vi "Util_GetLibraryVersion.vi"() -> (2 "TrajLibVersion":string)   [LabVIEW 2019, in "Trajectory_Library.lvlib"]
doc: "Return the library Trajectory Library version string.\n\n\n\nCopyright (c) 2020 James A. Simpson\nAll rights reserved.\n\nRedistribution and use in source and binary forms, with or without\nmodification, are permitted provided that the following conditions are met:\n * Redistributions of source code must retain the above copyright\n notice, this list of conditions and the following disclaimer.\n * Redistributions in binary form must reproduce the above copyright\n notice, this list of conditions and the following disclaimer in the\n documentation and/or other materials provided with the distribution.\n * Neither the name of the authors nor the\n names of its contributors may be used to endorse or promote products\n derived from this software without specific prior written permission.\n\nTHIS SOFTWARE IS PROVIDED BY THE AUTHOR AND CONTRIBUTORS``AS IS'' AND ANY\nEXPRESS OR IMPLIED WARRANTIES, INCLUDING, BUT NOT LIMITED TO, THE IMPLIED\nWARRANTIES OF MERCHANTABILITY NONINFRINGEMENT AND FITNESS FOR A PARTICULAR\nPURPOSE ARE DISCLAIMED. IN NO EVENT SHALL AUTHORS OR CONTRIBUTORS BE LIABLE FOR\nANY DIRECT, INDIRECT, INCIDENTAL, SPECIAL, EXEMPLARY, OR CONSEQUENTIAL DAMAGES\n(INCLUDING, BUT NOT LIMITED TO, PROCUREMENT OF SUBSTITUTE GOODS OR SERVICES;\nLOSS OF USE, DATA, OR PROFITS; OR BUSINESS INTERRUPTION) HOWEVER CAUSED AND\nON ANY THEORY OF LIABILITY, WHETHER IN CONTRACT, STRICT LIABILITY, OR TORT\n(INCLUDING NEGLIGENCE OR OTHERWISE) ARISING IN ANY WAY OUT OF THE USE OF THIS\nSOFTWARE, EVEN IF ADVISED OF THE POSSIBILITY OF SUCH DAMAGE.\n\n---------------------------------------------------------------------------------------------------\n==============================================================================\nCopyrights and Licenses for Third Party Software Distributed with FRC LV TRAJECTORY LIbrary\n==============================================================================\nThe FRC LV Trajectory Library software contains code written by and derived from \nthird parties. The copyrights, license, and restrictions which apply to each piece \nof software is included later in this file and/or inside of the individual \napplicable source files.\n\nThe disclaimer of warranty in the FRC LV Trajectory Library license above applies \nto all code in FRC LV Trajectory Library, and nothing in any of the other licenses \ngives permission to use the names of FIRST nor the names of the FRC LV Trajectory \nLibrary contributors to endorse or promote products derived from this software.\n\nThe following pieces of software have additional or alternate copyrights,\nlicenses, and/or restrictions:\n\nProgram Locations\n------- ---------\nWPILIB LabVIEW code derived from WPILIB\nRoboRIO Libraries ni-libraries\nPathfinder Pathfinder Library\nJSON for Modern C++ LabVIEW code derived from WPILIB routines\nTeam 254 Library LabVIEW code derived from WPILIB SplineParameterizer.java, \n TrajectoryParameterizer.java\n\n==============================================================================\nWPILIB License\n==============================================================================\nCopyright (c) 2009-2018 FIRST\nAll rights reserved.\n\nRedistribution and use in source and binary forms, with or without\nmodification, are permitted provided that the following conditions are met:\n * Redistributions of source code must retain the above copyright\n notice, this list of conditions and the following disclaimer.\n * Redistributions in binary form must reproduce the above copyright\n notice, this list of conditions and the following disclaimer in the\n documentation and/or other materials provided with the distribution.\n * Neither the name of the FIRST nor the\n names of its contributors may be used to endorse or promote products\n derived from this software without specific prior written permission.\n\nTHIS SOFTWARE IS PROVIDED BY FIRST AND CONTRIBUTORS``AS IS'' AND ANY\nEXPRESS OR IMPLIED WARRANTIES, INCLUDING, BUT NOT LIMITED TO, THE IMPLIED\nWARRANTIES OF MERCHANTABILITY NONINFRINGEMENT AND FITNESS FOR A PARTICULAR\nPURPOSE ARE DISCLAIMED. IN NO EVENT SHALL FIRST OR CONTRIBUTORS BE LIABLE FOR\nANY DIRECT, INDIRECT, INCIDENTAL, SPECIAL, EXEMPLARY, OR CONSEQUENTIAL DAMAGES\n(INCLUDING, BUT NOT LIMITED TO, PROCUREMENT OF SUBSTITUTE GOODS OR SERVICES;\nLOSS OF USE, DATA, OR PROFITS; OR BUSINESS INTERRUPTION) HOWEVER CAUSED AND\nON ANY THEORY OF LIABILITY, WHETHER IN CONTRACT, STRICT LIABILITY, OR TORT\n(INCLUDING NEGLIGENCE OR OTHERWISE) ARISING IN ANY WAY OUT OF THE USE OF THIS\nSOFTWARE, EVEN IF ADVISED OF THE POSSIBILITY OF SUCH DAMAGE.\n\n==============================================================================\nPATHFINDER License\n==============================================================================\nThe MIT License (MIT)\n\nCopyright (c) 2016 Jaci R\n\nPermission is hereby granted, free of charge, to any person obtaining a copy\nof this software and associated documentation files (the \"Software\"), to deal\nin the Software without restriction, including without limitation the rights\nto use, copy, modify, merge, publish, distribute, sublicense, and/or sell\ncopies of the Software, and to permit persons to whom the Software is\nfurnished to do so, subject to the following conditions:\n\nThe above copyright notice and this permission notice shall be included in all\ncopies or substantial portions of the Software.\n\nTHE SOFTWARE IS PROVIDED \"AS IS\", WITHOUT WARRANTY OF ANY KIND, EXPRESS OR\nIMPLIED, INCLUDING BUT NOT LIMITED TO THE WARRANTIES OF MERCHANTABILITY,\nFITNESS FOR A PARTICULAR PURPOSE AND NONINFRINGEMENT. IN NO EVENT SHALL THE\nAUTHORS OR COPYRIGHT HOLDERS BE LIABLE FOR ANY CLAIM, DAMAGES OR OTHER\nLIABILITY, WHETHER IN AN ACTION OF CONTRACT, TORT OR OTHERWISE, ARISING FROM,\nOUT OF OR IN CONNECTION WITH THE SOFTWARE OR THE USE OR OTHER DEALINGS IN THE\nSOFTWARE.\n\n==============================================================================\nJSON for Modern C++ License\n==============================================================================\n\n __ _____ _____ _____\n __| | __| | | | JSON for Modern C++\n| | |__ | | | | | | version 2.1.1\n|_____|_____|_____|_|___| https://github.com/nlohmann/json\n\nLicensed under the MIT License <http://opensource.org/licenses/MIT>.\nCopyright (c) 2013-2017 Niels Lohmann <http://nlohmann.me>.\n\nPermission is hereby granted, free of charge, to any person obtaining a copy\nof this software and associated documentation files (the \"Software\"), to deal\nin the Software without restriction, including without limitation the rights\nto use, copy, modify, merge, publish, distribute, sublicense, and/or sell\ncopies of the Software, and to permit persons to whom the Software is\nfurnished to do so, subject to the following conditions:\n\nThe above copyright notice and this permission notice shall be included in all\ncopies or substantial portions of the Software.\n\nTHE SOFTWARE IS PROVIDED \"AS IS\", WITHOUT WARRANTY OF ANY KIND, EXPRESS OR\nIMPLIED, INCLUDING BUT NOT LIMITED TO THE WARRANTIES OF MERCHANTABILITY,\nFITNESS FOR A PARTICULAR PURPOSE AND NONINFRINGEMENT. IN NO EVENT SHALL THE\nAUTHORS OR COPYRIGHT HOLDERS BE LIABLE FOR ANY CLAIM, DAMAGES OR OTHER\nLIABILITY, WHETHER IN AN ACTION OF CONTRACT, TORT OR OTHERWISE, ARISING FROM,\nOUT OF OR IN CONNECTION WITH THE SOFTWARE OR THE USE OR OTHER DEALINGS IN THE\nSOFTWARE.\n\n\n\n\n================\nTeam 254 Library\n================\nMIT License\n\nCopyright (c) 2018 Team 254\n\nPermission is hereby granted, free of charge, to any person obtaining a copy\nof this software and associated documentation files (the \"Software\"), to deal\nin the Software without restriction, including without limitation the rights\nto use, copy, modify, merge, publish, distribute, sublicense, and/or sell\ncopies of the Software, and to permit persons to whom the Software is\nfurnished to do so, subject to the following conditions:\n\nThe above copyright notice and this permission notice shall be included in all\ncopies or substantial portions of the Software.\n\nTHE SOFTWARE IS PROVIDED \"AS IS\", WITHOUT WARRANTY OF ANY KIND, EXPRESS OR\nIMPLIED, INCLUDING BUT NOT LIMITED TO THE WARRANTIES OF MERCHANTABILITY,\nFITNESS FOR A PARTICULAR PURPOSE AND NONINFRINGEMENT. IN NO EVENT SHALL THE\nAUTHORS OR COPYRIGHT HOLDERS BE LIABLE FOR ANY CLAIM, DAMAGES OR OTHER\nLIABILITY, WHETHER IN AN ACTION OF CONTRACT, TORT OR OTHERWISE, ARISING FROM,\nOUT OF OR IN CONNECTION WITH THE SOFTWARE OR THE USE OR OTHER DEALINGS IN THE\nSOFTWARE."
uses:
  Trajectory_Library.lvlib
panel:
  # "Copyright (c) 2020 James A. Simpson\nAll rights reserved.\n\nRedistribution and use in source and binary forms, with or without\nmodification, are permitted provided that the following conditions are met:\n    * Redistributions of source code must retain the above copyright\n      notice, this list of conditions and the following disclaimer.\n    * Redistributions in binary form must reproduce the above copyright\n      notice, this list of conditions and the following disclaimer in the\n      documentation and/or other materials provided with the distribution.\n    * Neither the name of the authors nor the\n      names of its contributors may be used to endorse or promote products\n      derived from this software without specific prior written permission.\n\nTHIS SOFTWARE IS PROVIDED BY THE AUTHOR AND CONTRIBUTORS``AS IS'' AND ANY\nEXPRESS OR IMPLIED WARRANTIES, INCLUDING, BUT NOT LIMITED TO, THE IMPLIED\nWARRANTIES OF MERCHANTABILITY NONINFRINGEMENT AND FITNESS FOR A PARTICULAR\nPURPOSE ARE DISCLAIMED. IN NO EVENT SHALL AUTHORS OR CONTRIBUTORS BE LIABLE FOR\nANY DIRECT, INDIRECT, INCIDENTAL, SPECIAL, EXEMPLARY, OR CONSEQUENTIAL DAMAGES\n(INCLUDING, BUT NOT LIMITED TO, PROCUREMENT OF SUBSTITUTE GOODS OR SERVICES;\nLOSS OF USE, DATA, OR PROFITS; OR BUSINESS INTERRUPTION) HOWEVER CAUSED AND\nON ANY THEORY OF LIABILITY, WHETHER IN CONTRACT, STRICT LIABILITY, OR TORT\n(INCLUDING NEGLIGENCE OR OTHERWISE) ARISING IN ANY WAY OUT OF THE USE OF THIS\nSOFTWARE, EVEN IF ADVISED OF THE POSSIBILITY OF SUCH DAMAGE.\n\n---------------------------------------------------------------------------------------------------\n==============================================================================\nCopyrights and Licenses for Third Party Software Distributed with FRC LV TRAJECTORY LIbrary\n==============================================================================\nThe FRC LV Trajectory Library software contains code written by and derived from \nthird parties.  The copyrights, license, and restrictions which apply to each piece \nof software is included later in this file and/or inside of the individual \napplicable source files.\n\nThe disclaimer of warranty in the FRC LV Trajectory Library license above applies \nto all code in FRC LV Trajectory Library, and nothing in any of the other licenses \ngives permission to use the names of FIRST nor the names of the FRC LV Trajectory \nLibrary contributors to endorse or promote products derived from this software.\n\nThe following pieces of software have additional or alternate copyrights,\nlicenses, and/or restrictions:\n\nProgram               Locations\n-------               ---------\nWPILIB                LabVIEW code derived from WPILIB\nRoboRIO Libraries     ni-libraries\nPathfinder            Pathfinder Library\nJSON for Modern C++   LabVIEW code derived from WPILIB routines\nTeam 254 Library      LabVIEW code derived from WPILIB SplineParameterizer.java, \n                      TrajectoryParameterizer.java\n\n==============================================================================\nWPILIB License\n==============================================================================\nCopyright (c) 2009-2018 FIRST\nAll rights reserved.\n\nRedistribution and use in source and binary forms, with or without\nmodification, are permitted provided that the following conditions are met:\n    * Redistributions of source code must retain the above copyright\n      notice, this list of conditions and the following disclaimer.\n    * Redistributions in binary form must reproduce the above copyright\n      notice, this list of conditions and the following disclaimer in the\n      documentation and/or other materials provided with the distribution.\n    * Neither the name of the FIRST nor the\n      names of its contributors may be used to endorse or promote products\n      derived from this software without specific prior written permission.\n\nTHIS SOFTWARE IS PROVIDED BY FIRST AND CONTRIBUTORS``AS IS'' AND ANY\nEXPRESS OR IMPLIED WARRANTIES, INCLUDING, BUT NOT LIMITED TO, THE IMPLIED\nWARRANTIES OF MERCHANTABILITY NONINFRINGEMENT AND FITNESS FOR A PARTICULAR\nPURPOSE ARE DISCLAIMED. IN NO EVENT SHALL FIRST OR CONTRIBUTORS BE LIABLE FOR\nANY DIRECT, INDIRECT, INCIDENTAL, SPECIAL, EXEMPLARY, OR CONSEQUENTIAL DAMAGES\n(INCLUDING, BUT NOT LIMITED TO, PROCUREMENT OF SUBSTITUTE GOODS OR SERVICES;\nLOSS OF USE, DATA, OR PROFITS; OR BUSINESS INTERRUPTION) HOWEVER CAUSED AND\nON ANY THEORY OF LIABILITY, WHETHER IN CONTRACT, STRICT LIABILITY, OR TORT\n(INCLUDING NEGLIGENCE OR OTHERWISE) ARISING IN ANY WAY OUT OF THE USE OF THIS\nSOFTWARE, EVEN IF ADVISED OF THE POSSIBILITY OF SUCH DAMAGE.\n\n==============================================================================\nPATHFINDER License\n==============================================================================\nThe MIT License (MIT)\n\nCopyright (c) 2016 Jaci R\n\nPermission is hereby granted, free of charge, to any person obtaining a copy\nof this software and associated documentation files (the \"Software\"), to deal\nin the Software without restriction, including without limitation the rights\nto use, copy, modify, merge, publish, distribute, sublicense, and/or sell\ncopies of the Software, and to permit persons to whom the Software is\nfurnished to do so, subject to the following conditions:\n\nThe above copyright notice and this permission notice shall be included in all\ncopies or substantial portions of the Software.\n\nTHE SOFTWARE IS PROVIDED \"AS IS\", WITHOUT WARRANTY OF ANY KIND, EXPRESS OR\nIMPLIED, INCLUDING BUT NOT LIMITED TO THE WARRANTIES OF MERCHANTABILITY,\nFITNESS FOR A PARTICULAR PURPOSE AND NONINFRINGEMENT. IN NO EVENT SHALL THE\nAUTHORS OR COPYRIGHT HOLDERS BE LIABLE FOR ANY CLAIM, DAMAGES OR OTHER\nLIABILITY, WHETHER IN AN ACTION OF CONTRACT, TORT OR OTHERWISE, ARISING FROM,\nOUT OF OR IN CONNECTION WITH THE SOFTWARE OR THE USE OR OTHER DEALINGS IN THE\nSOFTWARE.\n\n==============================================================================\nJSON for Modern C++ License\n==============================================================================\n\n    __ _____ _____ _____\n __|  |   __|     |   | |  JSON for Modern C++\n|  |  |__   |  |  | | | |  version 2.1.1\n|_____|_____|_____|_|___|  https://github.com/nlohmann/json\n\nLicensed under the MIT License <http://opensource.org/licenses/MIT>.\nCopyright (c) 2013-2017 Niels Lohmann <http://nlohmann.me>.\n\nPermission is hereby  granted, free of charge, to any  person obtaining a copy\nof this software and associated  documentation files (the \"Software\"), to deal\nin the Software  without restriction, including without  limitation the rights\nto  use, copy,  modify, merge,  publish, distribute,  sublicense, and/or  sell\ncopies  of  the Software,  and  to  permit persons  to  whom  the Software  is\nfurnished to do so, subject to the following conditions:\n\nThe above copyright notice and this permission notice shall be included in all\ncopies or substantial portions of the Software.\n\nTHE SOFTWARE  IS PROVIDED \"AS  IS\", WITHOUT WARRANTY  OF ANY KIND,  EXPRESS OR\nIMPLIED,  INCLUDING BUT  NOT  LIMITED TO  THE  WARRANTIES OF  MERCHANTABILITY,\nFITNESS FOR  A PARTICULAR PURPOSE AND  NONINFRINGEMENT. IN NO EVENT  SHALL THE\nAUTHORS  OR COPYRIGHT  HOLDERS  BE  LIABLE FOR  ANY  CLAIM,  DAMAGES OR  OTHER\nLIABILITY, WHETHER IN AN ACTION OF  CONTRACT, TORT OR OTHERWISE, ARISING FROM,\nOUT OF OR IN CONNECTION WITH THE SOFTWARE  OR THE USE OR OTHER DEALINGS IN THE\nSOFTWARE.\n\n\n\n\n================\nTeam 254 Library\n================\nMIT License\n\nCopyright (c) 2018 Team 254\n\nPermission is hereby granted, free of charge, to any person obtaining a copy\nof this software and associated documentation files (the \"Software\"), to deal\nin the Software without restriction, including without limitation the rights\nto use, copy, modify, merge, publish, distribute, sublicense, and/or sell\ncopies of the Software, and to permit persons to whom the Software is\nfurnished to do so, subject to the following conditions:\n\nThe above copyright notice and this permission notice shall be included in all\ncopies or substantial portions of the Software.\n\nTHE SOFTWARE IS PROVIDED \"AS IS\", WITHOUT WARRANTY OF ANY KIND, EXPRESS OR\nIMPLIED, INCLUDING BUT NOT LIMITED TO THE WARRANTIES OF MERCHANTABILITY,\nFITNESS FOR A PARTICULAR PURPOSE AND NONINFRINGEMENT. IN NO EVENT SHALL THE\nAUTHORS OR COPYRIGHT HOLDERS BE LIABLE FOR ANY CLAIM, DAMAGES OR OTHER\nLIABILITY, WHETHER IN AN ACTION OF CONTRACT, TORT OR OTHERWISE, ARISING FROM,\nOUT OF OR IN CONNECTION WITH THE SOFTWARE OR THE USE OR OTHER DEALINGS IN THE\nSOFTWARE."
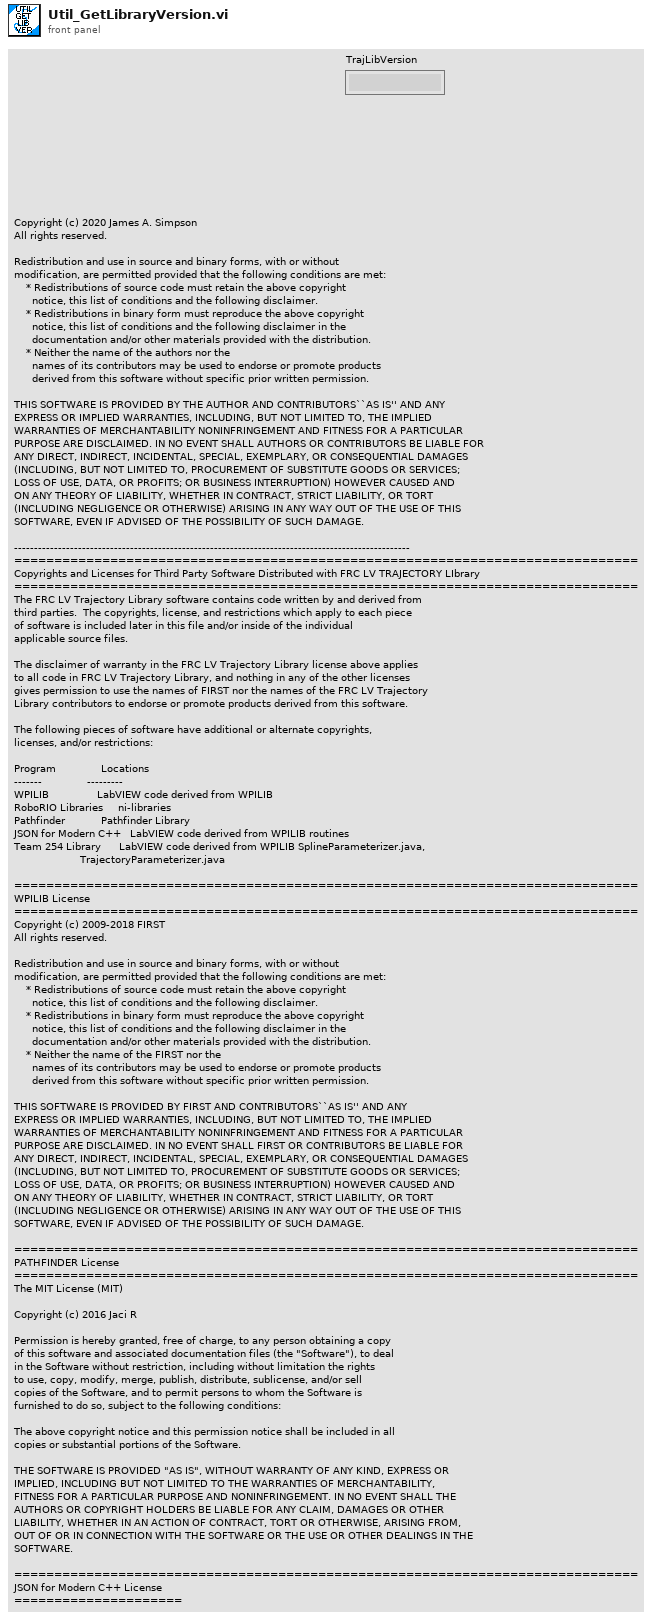
[diagram p1: front panel]
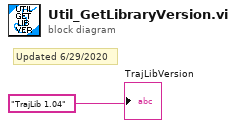
[diagram p0: block diagram]
diagram:
  # "Updated 6/29/2020"
  "TrajLibVersion" <- "TrajLib 1.04" ("TrajLibVersion")
